vi "SentinelController v33.vi"() -> ()   [LabVIEW 2011] (continued)
                                n1665 = local write "GPIB bus 0 write error"(w1891) -> ()
                                n1666 = local write "GPIB Bus 0 traffic"(w1885) -> ()
                                }
                                }
                                frame #2 {
                                n1667 = local read "H2 loop counter hid"() -> (w1892:u32)
                                n1668 = Increment(x=w1892) -> (x+1=w1893:u32)
                                n1669 = local write "H2 loop counter hid"(w1893) -> ()
                                }
                                }
                                }
                                }
                                }
                                frame True {
                                n1670 = flat-sequence {
                                frame #0 {
                                n1671 = local write "Last locked handler hid"(enum16{"H1", "H2"}."H1" ("Last locked handler")) -> ()
                                }
                                frame #1 {
                                n1672 = while {
                                stop <- w1895 stop-if-true
                                n1673 = local read "VISA bus 0 resource name out hid"() -> (w1904:refnum<visa-resource-name>)
                                n1674 = local read "H1 SITES? response hid"() -> (w1898:string)
                                n1675 = local read "VISA bus 0 error out hid"() -> (w1905:errorcluster)
                                n1676 = VISA Write(VISA resource name=w1904, write buffer=w1898, error in (no error)=w1905) -> (VISA resource name out=w1903:refnum<visa-resource-name>, return count=w1896:u32, error out=w1902:errorcluster)
                                n1677 = local write "VISA bus 0 resource name out hid"(w1903) -> ()
                                n1678 = local write "VISA bus 0 error out hid"(w1902) -> ()
                                n1679 = Unbundle By Name(w1902) -> ("status"=w1906:bool)
                                n1680 = Concatenate Strings("H1: Tester test cycle start" ("string"), "\r\n", "Bus 0 write: " ("string"), w1898) -> (w1900:string)
                                n1681 = Greater Than 0?(x=w1896) -> (x > 0?=w1895:bool)
                                n1682 = local write "GPIB bus 0 write error"(w1906) -> ()
                                n1683 = local write "GPIB Bus 0 traffic"(w1900) -> ()
                                }
                                }
                                frame #2 {
                                n1684 = local read "H1 loop counter hid"() -> (w1908:u32)
                                n1685 = Increment(x=w1908) -> (x+1=w1907:u32)
                                n1686 = local write "H1 loop counter hid"(w1907) -> ()
                                }
                                }
                                }
                                }
                                }
                                }
                                }
                                frame #2 {
                                n1687 = Tick Count (ms)() -> (millisecond timer value=w1911:u32)
                                n1688 = Tick Count (ms)() -> (millisecond timer value=w1912:u32)
                                n1689 = local write "tester tt start hid"(w1911) -> ()
                                n1690 = local write "tester wt end hid"(w1912) -> ()
                                }
                                frame #3 {
                                n1691 = local read "tester wt start hid"() -> (w1916:u32)
                                n1692 = local read "tester wt end hid"() -> (w1917:u32)
                                n1693 = Subtract(x=w1917, y=w1916) -> (x-y=w1915:u32)
                                n1694 = Divide(x=w1915, y=u32 1000) -> (x/y=w1913:dbl)
                                n1695 = local write "SC measured wait time hid"(w1913) -> ()
                                }
                                frame #4 {
                                n1696 = local write "SC handler states hid"(SC_handler_states."testing" ("SC Test Interface States")) -> ()
                                }
                                }
                                }
                                }
                              }
                              frame "testing" {
                                n1697 = flat-sequence {
                                frame #0 {
                                # "Why not just go back to \"waiting on event\" state?  BEcause the state machine needs\nto sequence to a \"testing state\" so that the user knows where the program is and\nso that the monitor can show this as the current state... which is what it is.  So\nthis state is equivalent to the \"waiting on event\" state.  It is just called \"testing.\"\nA binning event will exit this state and take it to the \"reading\" state."
                                }
                                frame #1 {
                                n1698 = local read "VISA bus 0 resource name out hid"() -> (w1929:refnum<visa-resource-name>)
                                n1699 = local read "VISA bus 0 error out hid"() -> (w1928:errorcluster)
                                n1700 = local read "GPIB wait timeout hid"() -> (w1925:u32)
                                n1701 = VISA Wait on Event(7:w1925, 8:w1928, 11:w1929) -> (0:w1926:errorcluster, 3:w1927:refnum<visa-resource-name>)  [unwired: 2 in, 2 out]
                                n1702 = local write "VISA bus 0 resource name out hid"(w1927) -> ()
                                n1703 = local write "VISA bus 0 error out hid"(w1926) -> ()
                                }
                                frame #2 {
                                n1704 = local read "Tester loop counter hid"() -> (w1930:u32)
                                n1705 = Increment(x=w1930) -> (x+1=w1931:u32)
                                n1706 = local write "Tester loop counter hid"(w1931) -> ()
                                }
                                frame #3 {
                                n1707 = local write "SC handler states hid"(SC_handler_states."reading" ("SC Test Interface States")) -> ()
                                }
                                }
                              }
                              frame "responding to A BIN" {
                                n1708 = flat-sequence {
                                frame #0 {
                                n1709 = local read "H1 Lock"() -> (w1935:bool)
                                n1710 = case shown="False" w1935 {
                                frame False {
                                n1711 = local read "H2 Lock"() -> (w1936:bool)
                                n1712 = case shown="True" w1936 {
                                frame False {
                                }
                                frame True {
                                n1713 = local read "GPIB Bus 0 traffic"() -> (w1940:string)
                                n1714 = Concatenate Strings(w1940, "\r\n", "Bus 0: binning, calulating\ntest time, financials, releasing\nH2 lock." ("string")) -> (w1938:string)
                                n1715 = local write "GPIB Bus 0 traffic"(w1938) -> ()
                                }
                                }
                                }
                                frame True {
                                n1716 = local read "GPIB Bus 0 traffic"() -> (w1944:string)
                                n1717 = Concatenate Strings(w1944, "\r\n", "Bus 0: binning, calulating\ntest time, financials, releasing\nH1 lock." ("string")) -> (w1942:string)
                                n1718 = local write "GPIB Bus 0 traffic"(w1942) -> ()
                                }
                                }
                                }
                                frame #1 {
                                n1719 = Tick Count (ms)() -> (millisecond timer value=w1946:u32)
                                n1720 = Tick Count (ms)() -> (millisecond timer value=w1945:u32)
                                n1721 = local write "tester tt end hid"(w1946) -> ()
                                n1722 = local write "tester wt start hid"(w1945) -> ()
                                }
                                frame #2 {
                                n1723 = local read "tester tt start hid"() -> (w1950:u32)
                                n1724 = local read "tester tt end hid"() -> (w1951:u32)
                                n1725 = Subtract(x=w1951, y=w1950) -> (x-y=w1949:u32)
                                n1726 = Divide(x=w1949, y=u32 1000) -> (x/y=w1947:dbl)
                                n1727 = local write "SC measured test time hid"(w1947) -> ()
                                }
                                frame #3 {
                                n1728 = local read "H1 Lock"() -> (w1952:bool)
                                n1729 = case shown="True" w1952 {
                                frame False {
                                n1730 = local read "H2 Lock"() -> (w1953:bool)
                                n1731 = case shown="True" w1953 {
                                frame False {
                                n1732 = One Button Dialog(message="Fatal error 202:\nThe SC responded to a handler being ready with devices\nto test, but when the SC received binning data, no handler had a lock. \nPlease report this bug to Celerint at www.celerint.com  ") -> ()  [unwired: 1 in, 1 out]
                                }
                                frame True {
                                n1733 = local read "H2 online"() -> (w1974:bool)
                                n1734 = local read "Tandem\nfloorspace area"() -> (w1957:i32)
                                n1735 = local read "Std cell \nfloorspace area"() -> (w1985:i32)
                                n1736 = case shown="True" w1974 {
                                tunnel: [0 w1989] -> w1975
                                frame False {
                                }
                                frame True {
                                n1737 = local read "H2 UPH"() -> (w1990:cluster{u32, u32})
                                n1738 = Unbundle(w1990) -> (w1989:u32)  [unwired: 1 out]
                                }
                                }
                                n1739 = local read "System UPH"() -> (w1956:u32)
                                n1740 = local read "UPH"() -> (w1986:dbl)
                                n1741 = Divide(x=w1956, y=w1957) -> (x/y=w1955:dbl)
                                n1742 = local write "Tandem UPH\nper unit area"(w1955) -> ()
                                n1743 = Divide(x=w1986, y=w1985) -> (x/y=w1987:dbl)
                                n1744 = local read "Std hourly\ncost ($/hr)"() -> (w1982:dbl)
                                n1745 = local read "H1 UPH"() -> (w1984:cluster{u32, u32})
                                n1746 = local write "H1 UPH per unit area"(w1987) -> ()
                                n1747 = local read "Utilization (%)"() -> (w1967:u32)
                                n1748 = local read "Tandem hourly\ncost ($/hr)"() -> (w1983:dbl)
                                n1749 = local read "# of devices to test"() -> (w1973:u32)
                                n1750 = Unbundle(w1984) -> (w1976:u32)  [unwired: 1 out]
                                n1751 = local read "Hours per month"() -> (w1968:i32)
                                n1752 = local write "Calc H2 UPH"(w1975) -> ()
                                n1753 = local write "Calc H1 UPH"(w1976) -> ()
                                n1754 = local read "UPH"() -> (w1981:dbl)
                                n1755 = Add(x=w1976, y=w1975) -> (x+y=w1963:u32)
                                n1756 = Divide(x=w1967, y=u32 100) -> (x/y=w1966:dbl)
                                n1757 = Divide(x=w1973, y=w1963) -> (x/y=w1972:dbl)
                                n1758 = Multiply(x=w1968, y=w1966) -> (x*y=w1964:dbl)
                                n1759 = Divide(x=w1982, y=w1981) -> (x/y=w1980:dbl)
                                n1760 = Divide(x=w1983, y=w1963) -> (x/y=w1978:dbl)
                                n1761 = local write "System UPH"(w1963) -> ()
                                n1762 = local write "Calc\nsystem UPH"(w1963) -> ()
                                n1763 = local read "# of devices to test"() -> (w1961:u32)
                                n1764 = Divide(x=w1972, y=w1964) -> (x/y=w1971:dbl)
                                n1765 = Multiply(x=w1980, y=100.0) -> (x*y=w1959:dbl)
                                n1766 = Multiply(x=w1978, y=100.0) -> (x*y=w1958:dbl)
                                n1767 = local write "Std unit cost\n(cents/device)"(w1959) -> ()
                                n1768 = local write "Tandem unit cost\n(cents/device)"(w1958) -> ()
                                n1769 = Subtract(x=w1959, y=w1958) -> (x-y=w1962:dbl)
                                n1770 = Multiply(x=w1971, y=30) -> (x*y=w1969:dbl)
                                n1771 = Multiply(x=w1961, y=w1962) -> (x*y=w1960:dbl)
                                n1772 = local write "Calendar days required\nfor testing all units"(w1969) -> ()
                                n1773 = local write "$ saved"(w1960) -> ()
                                }
                                }
                                }
                                frame True {
                                n1774 = local read "H1 online"() -> (w2011:bool)
                                n1775 = local read "Tandem\nfloorspace area"() -> (w2023:i32)
                                n1776 = local read "Std cell \nfloorspace area"() -> (w2016:i32)
                                n1777 = case shown="True" w2011 {
                                tunnel: [0 w2025] -> w1991
                                frame False {
                                }
                                frame True {
                                n1778 = local read "H1 UPH"() -> (w2026:cluster{u32, u32})
                                n1779 = Unbundle(w2026) -> (w2025:u32)  [unwired: 1 out]
                                }
                                }
                                n1780 = local read "System UPH"() -> (w2022:u32)
                                n1781 = local read "H2 calc UPH"() -> (w2017:dbl)
                                n1782 = Divide(x=w2022, y=w2023) -> (x/y=w1994:dbl)
                                n1783 = Divide(x=w2017, y=w2016) -> (x/y=w1995:dbl)
                                n1784 = local write "Tandem UPH\nper unit area"(w1994) -> ()
                                n1785 = local write "H2 UPH per unit area"(w1995) -> ()
                                n1786 = local read "Std hourly\ncost ($/hr)"() -> (w2019:dbl)
                                n1787 = local read "H2 UPH"() -> (w2021:cluster{u32, u32})
                                n1788 = local read "Utilization (%)"() -> (w2001:u32)
                                n1789 = local read "Tandem hourly\ncost ($/hr)"() -> (w2020:dbl)
                                n1790 = local read "# of devices to test"() -> (w2007:u32)
                                n1791 = local read "Hours per month"() -> (w2002:i32)
                                n1792 = Unbundle(w2021) -> (w1997:u32)  [unwired: 1 out]
                                n1793 = local write "Calc H1 UPH"(w1991) -> ()
                                n1794 = local write "Calc H2 UPH"(w1997) -> ()
                                n1795 = local read "UPH"() -> (w2018:dbl)
                                n1796 = Add(x=w1991, y=w1997) -> (x+y=w1996:u32)
                                n1797 = Divide(x=w2001, y=u32 100) -> (x/y=w2000:dbl)
                                n1798 = local write "System UPH"(w1996) -> ()
                                n1799 = local write "Calc\nsystem UPH"(w1996) -> ()
                                n1800 = Divide(x=w2007, y=w1996) -> (x/y=w2006:dbl)
                                n1801 = Multiply(x=w2002, y=w2000) -> (x*y=w1998:dbl)
                                n1802 = Divide(x=w2019, y=w2018) -> (x/y=w2015:dbl)
                                n1803 = Divide(x=w2020, y=w1996) -> (x/y=w2013:dbl)
                                n1804 = local read "# of devices to test"() -> (w2009:u32)
                                n1805 = Divide(x=w2006, y=w1998) -> (x/y=w2005:dbl)
                                n1806 = Multiply(x=w2015, y=100.0) -> (x*y=w1993:dbl)
                                n1807 = Multiply(x=w2013, y=100.0) -> (x*y=w1992:dbl)
                                n1808 = local write "Std unit cost\n(cents/device)"(w1993) -> ()
                                n1809 = local write "Tandem unit cost\n(cents/device)"(w1992) -> ()
                                n1810 = Subtract(x=w1993, y=w1992) -> (x-y=w2010:dbl)
                                n1811 = Multiply(x=w2005, y=30) -> (x*y=w2003:dbl)
                                n1812 = Multiply(x=w2009, y=w2010) -> (x*y=w2008:dbl)
                                n1813 = local write "Calendar days required\nfor testing all units"(w2003) -> ()
                                n1814 = local write "$ saved"(w2008) -> ()
                                }
                                }
                                }
                                frame #4 {
                                # "when this loop unlocks the handlers,\nthe handler interface loops are free to continue\nto send the binning information to their\nrespective handlers.  Each handler interface \nloop using the \"binning string hidden\" to do\nthis.  That is why, here, there is no writing of\nthe binning informatrion to a handler.  \nThat is done in the handler interface loops."
                                n1815 = local write "H1 Lock"(FALSE ("H1 Lock")) -> ()
                                n1816 = local write "H2 Lock"(FALSE ("H1 Lock")) -> ()
                                }
                                frame #5 {
                                n1817 = local read "Tester online"() -> (w2029:bool)
                                n1818 = local read "POWER"() -> (w2031:bool)
                                n1819 = Compound Arithmetic op=AND(w2029, w2031) -> (w2030:bool)
                                n1820 = case shown="True" w2030 {
                                frame False {
                                n1821 = local write "SC handler states hid"(SC_handler_states."closing bus" ("SC virtual handler states")) -> ()
                                }
                                frame True {
                                n1822 = local write "SC handler states hid"(SC_handler_states."waiting on event" ("SC virtual handler states")) -> ()
                                }
                                }
                                }
                                }
                              }
                              frame "responding to BINON" {
                                n1823 = local read "H1 Lock"() -> (w2034:bool)
                                n1824 = case shown="True" w2034 {
                                frame False {
                                n1825 = local read "H2 Lock"() -> (w2037:bool)
                                n1826 = case shown="True" w2037 {
                                frame False {
                                }
                                frame True {
                                n1827 = flat-sequence {
                                frame #0 {
                                n1828 = local read "H2 echo hid"() -> (w2038:string)
                                n1829 = local read "VISA bus 0 resource name out hid"() -> (w2047:refnum<visa-resource-name>)
                                n1830 = local read "VISA bus 0 error out hid"() -> (w2046:errorcluster)
                                n1831 = local read "GPIB Bus 0 traffic"() -> (w2043:string)
                                n1832 = VISA Write(VISA resource name=w2047, write buffer=w2038, error in (no error)=w2046) -> (VISA resource name out=w2045:refnum<visa-resource-name>, error out=w2044:errorcluster)  [unwired: 1 out]
                                n1833 = local write "VISA bus 0 resource name out hid"(w2045) -> ()
                                n1834 = Unbundle By Name(w2044) -> ("status"=w2039:bool)
                                n1835 = local write "VISA bus 0 error out hid"(w2044) -> ()
                                n1836 = Concatenate Strings(w2043, "\r\n", "Bus 0 write: " ("string"), w2038) -> (w2041:string)
                                n1837 = local write "GPIB Bus 0 traffic"(w2041) -> ()
                                n1838 = local write "GPIB bus 0 write error"(w2039) -> ()
                                }
                                frame #1 {
                                n1839 = local write "SC handler states hid"(SC_handler_states."waiting on event" ("SC Test Interface States")) -> ()
                                }
                                }
                                }
                                }
                                }
                                frame True {
                                n1840 = flat-sequence {
                                frame #0 {
                                n1841 = local read "H1 echo hid"() -> (w2049:string)
                                n1842 = local read "VISA bus 0 resource name out hid"() -> (w2058:refnum<visa-resource-name>)
                                n1843 = local read "VISA bus 0 error out hid"() -> (w2057:errorcluster)
                                n1844 = local read "GPIB Bus 0 traffic"() -> (w2054:string)
                                n1845 = VISA Write(VISA resource name=w2058, write buffer=w2049, error in (no error)=w2057) -> (VISA resource name out=w2056:refnum<visa-resource-name>, error out=w2055:errorcluster)  [unwired: 1 out]
                                n1846 = local write "VISA bus 0 resource name out hid"(w2056) -> ()
                                n1847 = Unbundle By Name(w2055) -> ("status"=w2050:bool)
                                n1848 = local write "VISA bus 0 error out hid"(w2055) -> ()
                                n1849 = Concatenate Strings(w2054, "\r\n", "Bus 0 write: " ("string"), w2049) -> (w2052:string)
                                n1850 = local write "GPIB Bus 0 traffic"(w2052) -> ()
                                n1851 = local write "GPIB bus 0 write error"(w2050) -> ()
                                }
                                frame #1 {
                                n1852 = local write "SC handler states hid"(SC_handler_states."waiting on event" ("SC Test Interface States")) -> ()
                                }
                                }
                                }
                                }
                              }
                              frame "responding to ECHONG" {
                                n1853 = flat-sequence {
                                frame #0 {
                                # "Echo was returned to the tester via the BINON state"
                                n1854 = local read "H1 Lock"() -> (w2062:bool)
                                n1855 = case shown="False" w2062 {
                                frame False {
                                n1856 = local read "H2 Lock"() -> (w2063:bool)
                                n1857 = case shown="True" w2063 {
                                frame False {
                                }
                                frame True {
                                n1858 = local read "GPIB Bus 0 traffic"() -> (w2067:string)
                                n1859 = Concatenate Strings(w2067, "\r\n", "Bus 0: ECHONG received for H2. Retrying." ("string")) -> (w2065:string)
                                n1860 = local write "GPIB Bus 0 traffic"(w2065) -> ()
                                }
                                }
                                }
                                frame True {
                                n1861 = local read "GPIB Bus 0 traffic"() -> (w2071:string)
                                n1862 = Concatenate Strings(w2071, "\r\n", "Bus 0: ECHONG received for H1. Retrying." ("string")) -> (w2069:string)
                                n1863 = local write "GPIB Bus 0 traffic"(w2069) -> ()
                                }
                                }
                                }
                                frame #1 {
                                n1864 = local write "SC handler states hid"(SC_handler_states."waiting on event" ("SC Test Interface States")) -> ()
                                }
                                }
                              }
                              frame "responding to ECHOOK" {
                                n1865 = flat-sequence {
                                frame #0 {
                                # "Echo was returned to the tester via the BINON state"
                                n1866 = local read "H1 Lock"() -> (w2075:bool)
                                n1867 = case shown="True" w2075 {
                                frame False {
                                n1868 = local read "H2 Lock"() -> (w2076:bool)
                                n1869 = case shown="False" w2076 {
                                frame False {
                                }
                                frame True {
                                n1870 = local read "GPIB Bus 0 traffic"() -> (w2080:string)
                                n1871 = Concatenate Strings(w2080, "\r\n", "Bus 0: ECHOOK received for H2.\nCalculating test time, financials,\nreleasing H2 Lock." ("string")) -> (w2078:string)
                                n1872 = local write "GPIB Bus 0 traffic"(w2078) -> ()
                                }
                                }
                                }
                                frame True {
                                n1873 = local read "GPIB Bus 0 traffic"() -> (w2084:string)
                                n1874 = Concatenate Strings(w2084, "\r\n", "Bus 0: ECHOOK received for H1.\nCalculating test time, financials,\nreleasing H1 Lock." ("string")) -> (w2082:string)
                                n1875 = local write "GPIB Bus 0 traffic"(w2082) -> ()
                                }
                                }
                                }
                                frame #1 {
                                n1876 = Tick Count (ms)() -> (millisecond timer value=w2086:u32)
                                n1877 = Tick Count (ms)() -> (millisecond timer value=w2085:u32)
                                n1878 = local write "tester tt end hid"(w2086) -> ()
                                n1879 = local write "tester wt start hid"(w2085) -> ()
                                }
                                frame #2 {
                                n1880 = local read "tester tt start hid"() -> (w2090:u32)
                                n1881 = local read "tester tt end hid"() -> (w2091:u32)
                                n1882 = Subtract(x=w2091, y=w2090) -> (x-y=w2089:u32)
                                n1883 = Divide(x=w2089, y=u32 1000) -> (x/y=w2087:dbl)
                                n1884 = local write "SC measured test time hid"(w2087) -> ()
                                }
                                frame #3 {
                                n1885 = local read "H1 Lock"() -> (w2092:bool)
                                n1886 = case shown="True" w2092 {
                                frame False {
                                n1887 = local read "H2 Lock"() -> (w2093:bool)
                                n1888 = case shown="True" w2093 {
                                frame False {
                                n1889 = One Button Dialog(message="Fatal error 202:\nThe SC responded to a handler being ready with devices\nto test, but when the SC received binning data, no handler had a lock. \nPlease report this bug to Celerint at www.celerint.com  ") -> ()  [unwired: 1 in, 1 out]
                                }
                                frame True {
                                n1890 = local read "H2 online"() -> (w2114:bool)
                                n1891 = local read "Tandem\nfloorspace area"() -> (w2097:i32)
                                n1892 = local read "Std cell \nfloorspace area"() -> (w2125:i32)
                                n1893 = case shown="True" w2114 {
                                tunnel: [0 w2129] -> w2115
                                frame False {
                                }
                                frame True {
                                n1894 = local read "H2 UPH"() -> (w2130:cluster{u32, u32})
                                n1895 = Unbundle(w2130) -> (w2129:u32)  [unwired: 1 out]
                                }
                                }
                                n1896 = local read "System UPH"() -> (w2096:u32)
                                n1897 = local read "UPH"() -> (w2126:dbl)
                                n1898 = Divide(x=w2096, y=w2097) -> (x/y=w2095:dbl)
                                n1899 = local write "Tandem UPH\nper unit area"(w2095) -> ()
                                n1900 = Divide(x=w2126, y=w2125) -> (x/y=w2127:dbl)
                                n1901 = local read "Std hourly\ncost ($/hr)"() -> (w2122:dbl)
                                n1902 = local read "H1 UPH"() -> (w2124:cluster{u32, u32})
                                n1903 = local write "H1 UPH per unit area"(w2127) -> ()
                                n1904 = local read "Utilization (%)"() -> (w2107:u32)
                                n1905 = local read "Tandem hourly\ncost ($/hr)"() -> (w2123:dbl)
                                n1906 = local read "# of devices to test"() -> (w2113:u32)
                                n1907 = Unbundle(w2124) -> (w2116:u32)  [unwired: 1 out]
                                n1908 = local read "Hours per month"() -> (w2108:i32)
                                n1909 = local write "Calc H2 UPH"(w2115) -> ()
                                n1910 = local write "Calc H1 UPH"(w2116) -> ()
                                n1911 = local read "UPH"() -> (w2121:dbl)
                                n1912 = Add(x=w2116, y=w2115) -> (x+y=w2103:u32)
                                n1913 = Divide(x=w2107, y=u32 100) -> (x/y=w2106:dbl)
                                n1914 = Divide(x=w2113, y=w2103) -> (x/y=w2112:dbl)
                                n1915 = Multiply(x=w2108, y=w2106) -> (x*y=w2104:dbl)
                                n1916 = Divide(x=w2122, y=w2121) -> (x/y=w2120:dbl)
                                n1917 = Divide(x=w2123, y=w2103) -> (x/y=w2118:dbl)
                                n1918 = local write "System UPH"(w2103) -> ()
                                n1919 = local write "Calc\nsystem UPH"(w2103) -> ()
                                n1920 = local read "# of devices to test"() -> (w2101:u32)
                                n1921 = Divide(x=w2112, y=w2104) -> (x/y=w2111:dbl)
                                n1922 = Multiply(x=w2120, y=100.0) -> (x*y=w2099:dbl)
                                n1923 = Multiply(x=w2118, y=100.0) -> (x*y=w2098:dbl)
                                n1924 = local write "Std unit cost\n(cents/device)"(w2099) -> ()
                                n1925 = local write "Tandem unit cost\n(cents/device)"(w2098) -> ()
                                n1926 = Subtract(x=w2099, y=w2098) -> (x-y=w2102:dbl)
                                n1927 = Multiply(x=w2111, y=30) -> (x*y=w2109:dbl)
                                n1928 = Multiply(x=w2101, y=w2102) -> (x*y=w2100:dbl)
                                n1929 = local write "Calendar days required\nfor testing all units"(w2109) -> ()
                                n1930 = local write "$ saved"(w2100) -> ()
                                }
                                }
                                }
                                frame True {
                                n1931 = local read "H1 online"() -> (w2151:bool)
                                n1932 = local read "Tandem\nfloorspace area"() -> (w2163:i32)
                                n1933 = local read "Std cell \nfloorspace area"() -> (w2156:i32)
                                n1934 = case shown="True" w2151 {
                                tunnel: [0 w2165] -> w2131
                                frame False {
                                }
                                frame True {
                                n1935 = local read "H1 UPH"() -> (w2166:cluster{u32, u32})
                                n1936 = Unbundle(w2166) -> (w2165:u32)  [unwired: 1 out]
                                }
                                }
                                n1937 = local read "System UPH"() -> (w2162:u32)
                                n1938 = local read "H2 calc UPH"() -> (w2157:dbl)
                                n1939 = Divide(x=w2162, y=w2163) -> (x/y=w2134:dbl)
                                n1940 = Divide(x=w2157, y=w2156) -> (x/y=w2135:dbl)
                                n1941 = local write "Tandem UPH\nper unit area"(w2134) -> ()
                                n1942 = local write "H2 UPH per unit area"(w2135) -> ()
                                n1943 = local read "Std hourly\ncost ($/hr)"() -> (w2159:dbl)
                                n1944 = local read "H2 UPH"() -> (w2161:cluster{u32, u32})
                                n1945 = local read "Utilization (%)"() -> (w2141:u32)
                                n1946 = local read "Tandem hourly\ncost ($/hr)"() -> (w2160:dbl)
                                n1947 = local read "# of devices to test"() -> (w2147:u32)
                                n1948 = local read "Hours per month"() -> (w2142:i32)
                                n1949 = Unbundle(w2161) -> (w2137:u32)  [unwired: 1 out]
                                n1950 = local write "Calc H1 UPH"(w2131) -> ()
                                n1951 = local write "Calc H2 UPH"(w2137) -> ()
                                n1952 = local read "UPH"() -> (w2158:dbl)
                                n1953 = Add(x=w2131, y=w2137) -> (x+y=w2136:u32)
                                n1954 = Divide(x=w2141, y=u32 100) -> (x/y=w2140:dbl)
                                n1955 = local write "System UPH"(w2136) -> ()
                                n1956 = local write "Calc\nsystem UPH"(w2136) -> ()
                                n1957 = Divide(x=w2147, y=w2136) -> (x/y=w2146:dbl)
                                n1958 = Multiply(x=w2142, y=w2140) -> (x*y=w2138:dbl)
                                n1959 = Divide(x=w2159, y=w2158) -> (x/y=w2155:dbl)
                                n1960 = Divide(x=w2160, y=w2136) -> (x/y=w2153:dbl)
                                n1961 = local read "# of devices to test"() -> (w2149:u32)
                                n1962 = Divide(x=w2146, y=w2138) -> (x/y=w2145:dbl)
                                n1963 = Multiply(x=w2155, y=100.0) -> (x*y=w2133:dbl)
                                n1964 = Multiply(x=w2153, y=100.0) -> (x*y=w2132:dbl)
                                n1965 = local write "Std unit cost\n(cents/device)"(w2133) -> ()
                                n1966 = local write "Tandem unit cost\n(cents/device)"(w2132) -> ()
                                n1967 = Subtract(x=w2133, y=w2132) -> (x-y=w2150:dbl)
                                n1968 = Multiply(x=w2145, y=30) -> (x*y=w2143:dbl)
                                n1969 = Multiply(x=w2149, y=w2150) -> (x*y=w2148:dbl)
                                n1970 = local write "Calendar days required\nfor testing all units"(w2143) -> ()
                                n1971 = local write "$ saved"(w2148) -> ()
                                }
                                }
                                }
                                frame #4 {
                                # "when this loop unlocks the handlers,\nthe handler interface loops are free to continue\nto send the binning information to their\nrespective handlers.  Each handler interface \nloop using the \"binning string hidden\" to do\nthis.  That is why, here, there is no writing of\nthe binning informatrion to a handler.  \nThat is done in the handler interface loops."
                                n1972 = local write "H1 Lock"(FALSE ("H1 Lock")) -> ()
                                n1973 = local write "H2 Lock"(FALSE ("H1 Lock")) -> ()
                                }
                                frame #5 {
                                n1974 = local read "Tester online"() -> (w2169:bool)
                                n1975 = local read "POWER"() -> (w2171:bool)
                                n1976 = Compound Arithmetic op=AND(w2169, w2171) -> (w2170:bool)
                                n1977 = case shown="False" w2170 {
                                frame False {
                                n1978 = local write "SC handler states hid"(SC_handler_states."closing bus" ("SC virtual handler states")) -> ()
                                }
                                frame True {
                                n1979 = local write "SC handler states hid"(SC_handler_states."waiting on serial poll" ("SC Test Interface States")) -> ()
                                }
                                }
                                }
                                }
                              }
                              frame "closing bus" {
                                n1980 = flat-sequence {
                                frame #0 {
                                n1981 = local read "GPIB Bus 0 traffic"() -> (w2179:string)
                                n1982 = Concatenate Strings(w2179, "\r\n", "Bus 0 closing: " ("string")) -> (w2177:string)
                                n1983 = local write "GPIB Bus 0 traffic"(w2177) -> ()
                                }
                                frame #1 {
                                n1984 = local read "VISA bus 0 resource name out hid"() -> (w2181:refnum<visa-resource-name>)
                                n1985 = local read "VISA bus 0 error out hid"() -> (w2182:errorcluster)
                                n1986 = VISA Close(VISA resource name=w2181, error in (no error)=w2182) -> (error out=w2180:errorcluster)
                                n1987 = Unbundle By Name(w2180) -> ("status"=w2183:bool)
                                n1988 = local write "VISA bus 0 close error"(w2183) -> ()
                                }
                                frame #2 {
                                n1989 = local write "Exit SC handler StMach hid"(TRUE ("Exit tester state machine hid")) -> ()
                                }
                                }
                              }
                              frame "responding to unknown command" {
                                n1990 = flat-sequence {
                                frame #0 {
                                n1991 = local read "GPIB Bus 0 traffic"() -> (w2191:string)
                                n1992 = Concatenate Strings(w2191, "\r\n", "Bus 0 write: " ("string"), "unrecognized string") -> (w2189:string)
                                n1993 = local write "GPIB Bus 0 traffic"(w2189) -> ()
                                }
                                frame #1 {
                                n1994 = local write "SC handler states hid"(SC_handler_states."waiting on event" ("SC Test Interface States")) -> ()
                                }
                                }
                              }
                            }
                          }
                          frame #1 {
                            n1995 = local read "Slow for  Diagnostics"() -> (w2193:bool)
                            n1996 = case shown="True" w2193 {
                              frame False {
                              }
                              frame True {
                                n1997 = local read "GPIB wait time (ms)"() -> (w2196:u32)
                                n1998 = Wait (ms)(milliseconds to wait=w2196) -> ()  [unwired: 1 out]
                              }
                            }
                          }
                        }
                        n1999 = Wait (ms)(milliseconds to wait=u32 1) -> ()  [unwired: 1 out]
                        n2000 = local read "Exit SC handler StMach hid"() -> (w1380:bool)
                        "Numeric" <- w1376
                      }
                    }
                  }
                }
              }
              n2001 = Wait (ms)(milliseconds to wait=u32 5) -> ()  [unwired: 1 out]
              n2002 = local read "POWER"() -> (w1366:bool)
            }
            n2003 = while {
              stop <- w360 continue-if-true
              n2004 = local read "H1 online"() -> (w361:bool)
              n2005 = case shown="True" w361 {
                frame False {
                }
                frame True {
                  n2006 = flat-sequence {
                    frame #0 {
                      n2007 = local write "Exit SC tester H1 StMach hid"(FALSE ("Exit H1 state machine hid")) -> ()
                    }
                    frame #1 {
                      n2008 = local read "H1 handler type"() -> (w363:T2)
                      n2009 = case shown="\"Seiko-Epson NS6040\"" w363 {
                        frame "Multitest", Default {
                          n2010 = local write "MT99XX tester states H1 hid"(SC_MT99XX_tester_states."initializing bus" ("SC virtual tester states")) -> ()
                          n2011 = flat-sequence {
                            frame #0 {
                              n2012 = local read "MT99XX tester states H1 hid"() -> (w365:T4)
                              n2013 = case shown="\"binning\"" w365 {
                                frame "initializing bus", Default {
                                n2014 = flat-sequence {
                                frame #0 {
                                # "bus 1"
                                n2015 = local read "GPIB wait timeout hid"() -> (w369:u32)
                                n2016 = local read "SentCtrl talks to handler 1 at"() -> (w370:refnum<visa-resource-name>)
                                n2017 = local read "GPIB wait timeout hid"() -> (w368:u32)
                                n2018 = VISA Open(timeout (0)=w369, VISA resource name=w370) -> (VISA resource name=w367:refnum<visa-resource-name>, error out=w372:errorcluster)  [unwired: 3 in]
                                n2019 = property class="GPIB Instr"(reference=w367, error in=w372, "Timeout"=w368) -> (error out=w366:errorcluster)  [unwired: 1 out]
                                n2020 = local write "VISA bus 1 resource name out hid"(w367) -> ()
                                n2021 = Unbundle By Name(w366) -> ("status"=w371:bool)
                                n2022 = local write "VISA bus 1 open error"(w371) -> ()
                                n2023 = local write "VISA bus 1 error out hid"(w366) -> ()
                                }
                                frame #1 {
                                n2024 = local write "Exit SC tester H1 StMach hid"(FALSE ("Exit H1 state machine hid")) -> ()
                                n2025 = Concatenate Strings("Bus 1 initializing" ("string"), "\r\n") -> (w375:string)
                                n2026 = local write "GPIB bus 1 traffic"(w375) -> ()
                                }
                                frame #2 {
                                n2027 = local write "MT99XX tester states H1 hid"(SC_MT99XX_tester_states."sending *IDN?" ("SC virtual tester states")) -> ()
                                }
                                }
                                }
                                frame "sending *IDN?" {
                                n2028 = flat-sequence {
                                tunnel: [w387] -> w380
                                tunnel: [w386] -> w379
                                tunnel: w380 -> [w401]
                                tunnel: w379 -> [w400]
                                tunnel: [w391] -> w378
                                tunnel: w378 -> [w402]
                                frame #0 {
                                w381 = "*IDN?"
                                n2029 = local read "VISA bus 1 resource name out hid"() -> (w390:refnum<visa-resource-name>)
                                n2030 = local read "GPIB bus 1 traffic"() -> (w385:string)
                                n2031 = local read "VISA bus 1 error out hid"() -> (w389:errorcluster)
                                n2032 = Concatenate Strings(w385, "\r\n", "Bus 1 write: " ("string"), w381) -> (w383:string)
                                n2033 = VISA Write(VISA resource name=w390, write buffer=w381, error in (no error)=w389) -> (VISA resource name out=w387:refnum<visa-resource-name>, error out=w386:errorcluster)  [unwired: 1 out]
                                n2034 = Unbundle By Name(w386) -> ("status"=w388:bool)
                                n2035 = local write "GPIB bus 1 traffic"(w383) -> ()
                                n2036 = local write "GPIB bus 1 write error"(w388) -> ()
                                }
                                frame #1 {
                                n2037 = local read "GPIB bus 1 traffic"() -> (w393:string)
                                n2038 = VISA Read(VISA resource name=w401, byte count=u32 256, error in (no error)=w400) -> (VISA resource name out=w398:refnum<visa-resource-name>, read buffer=w392:string, error out=w397:errorcluster)  [unwired: 1 out]
                                n2039 = local write "VISA bus 1 resource name out hid"(w398) -> ()
                                n2040 = Unbundle By Name(w397) -> ("status"=w391:bool)
                                n2041 = local write "H1 response to *IDN? hid"(w392) -> ()
                                n2042 = local write "GPIB bus 1 read error"(w391) -> ()
                                n2043 = Concatenate Strings(w393, "\r\n", "Bus 1 read: " ("string"), w392) -> (w395:string)
                                n2044 = local write "GPIB bus 1 traffic"(w395) -> ()
                                }
                                frame #2 {
                                n2045 = case shown="False" w402 {
                                frame False {
                                n2046 = local write "MT99XX tester states H1 hid"(SC_MT99XX_tester_states."polling *SITES?" ("SC virtual tester states")) -> ()
                                }
                                frame True {
                                n2047 = flat-sequence {
                                frame #0 {
                                n2048 = while {
                                stop <- w405 stop-if-true
                                n2049 = One Button Dialog(message="Warning:\nVirtual tester does not get a response\nto *IDN? from handler 1.\nCheck GPIB cable and that  handler 1 \nis running and ready to issue a start of test\nby responding with sites ready.", button name ("OK")="Dismiss and retry") -> (true=w405:bool)
                                n2050 = Wait (ms)(milliseconds to wait=u32 100) -> ()  [unwired: 1 out]
                                }
                                }
                                frame #1 {
                                n2051 = local write "H1 online"(FALSE ("H1 online")) -> ()
                                }
                                frame #2 {
                                n2052 = local write "MT99XX tester states H1 hid"(SC_MT99XX_tester_states."sending *IDN?" ("SC virtual tester states")) -> ()
                                }
                                }
                                }
                                }
                                }
                                }
                                }
                                frame "polling *SITES?" {
                                n2053 = flat-sequence {
                                tunnel: [w413] -> w411
                                tunnel: [w412] -> w410
                                tunnel: w411 -> [w449]
                                tunnel: w410 -> [w448]
                                frame #0 {
                                n2054 = while {
                                tunnel: [w417] -> w413
                                tunnel: [w415] -> w412
                                stop <- w414 stop-if-true
                                n2055 = stacked-sequence {
                                tunnel: [w429] -> w419
                                tunnel: [w428] -> w418
                                frame #0 {
                                w421 = "*SITES?"
                                n2056 = local read "VISA bus 1 resource name out hid"() -> (w427:refnum<visa-resource-name>)
                                n2057 = local read "VISA bus 1 error out hid"() -> (w426:errorcluster)
                                n2058 = Concatenate Strings("Handler 1 cycle start" ("string"), "\r\n", "Bus 1 write: " ("string"), w421) -> (w423:string)
                                n2059 = VISA Write(VISA resource name=w427, write buffer=w421, error in (no error)=w426) -> (VISA resource name out=w429:refnum<visa-resource-name>, error out=w428:errorcluster)  [unwired: 1 out]
                                n2060 = Unbundle By Name(w428) -> ("status"=w425:bool)
                                n2061 = local write "GPIB bus 1 traffic"(w423) -> ()
                                n2062 = local write "GPIB bus 1 write error"(w425) -> ()
                                }
                                }
                                n2063 = Wait (ms)(milliseconds to wait=u32 1) -> ()  [unwired: 1 out]
                                n2064 = flat-sequence {
                                tunnel: w419 -> [w447]
                                tunnel: w418 -> [w446]
                                tunnel: [w434] -> w417
                                tunnel: [w430] -> w415
                                tunnel: [w431] -> w414
                                frame #0 {
                                n2065 = local read "GPIB bus 1 traffic"() -> (w439:string)
                                n2066 = VISA Read(VISA resource name=w447, byte count=u32 256, error in (no error)=w446) -> (read buffer=w434:string, error out=w433:errorcluster)  [unwired: 2 out]
                                n2067 = Unbundle By Name(w433) -> ("status"=w430:bool)
                                n2068 = String Length(string=w434) -> (length=w436:i32)
                                n2069 = Scan Value(string=w434, format string="%b", default (0 dbl)=u8 0) -> (value=w438:u8)  [unwired: 1 out]
                                n2070 = Concatenate Strings(w439, "\r\n", "Bus 1 read: " ("string"), w434) -> (w441:string)
                                n2071 = local write "GPIB bus 1 read error"(w430) -> ()
                                n2072 = Greater Than 0?(x=w436) -> (x > 0?=w435:bool)
                                n2073 = Greater Than 0?(x=w438) -> (x > 0?=w437:bool)
                                n2074 = local write "GPIB bus 1 traffic"(w441) -> ()
                                n2075 = And(x=w435, y=w437) -> (x .and. y?=w432:bool)
                                n2076 = Or(x=w432, y=w430) -> (x .or. y?=w431:bool)
                                }
                                }
                                }
                                }
                                frame #1 {
                                n2077 = case shown="False" w448 {
                                tunnel: w449 -> [w450 _]
                                frame False {
                                n2078 = flat-sequence {
                                tunnel: w450 -> [w451]
                                frame #0 {
                                n2079 = String Length(string=w451) -> (length=w452:i32)
                                n2080 = local write "H1 SITES? response hid"(w451) -> ()
                                n2081 = local write "H1 parallelism"(w452) -> ()
                                }
                                frame #1 {
                                # "This block adds zeroes (sites not ready)\nto SITES READY from handlers when the\nhandler is running at a lower parallelism\nthan the test program, but has the same\npin mapping for the active sites in common."
                                n2082 = local read "Program Parallelism"() -> (w456:u32)
                                n2083 = local read "H1 allow lower parallelism"() -> (w455:bool)
                                n2084 = local read "H1 parallelism"() -> (w457:u32)
                                n2085 = Less?(x=w457, y=w456) -> (x < y?=w454:bool)
                                n2086 = And(x=w454, y=w455) -> (x .and. y?=w453:bool)
                                n2087 = case shown="True" w453 {
                                frame False {
                                n2088 = local read "Program Parallelism"() -> (w460:u32)
                                n2089 = local read "H1 parallelism"() -> (w458:u32)
                                n2090 = Greater?(x=w458, y=w460) -> (0:w459:bool)
                                n2091 = case shown="True" w459 {
                                frame False {
                                # "parallelisms must match if arriving here"
                                n2092 = local write "MT99XX tester states H1 hid"(SC_MT99XX_tester_states."testing" ("SC virtual tester states")) -> ()
                                }
                                frame True {
                                n2093 = local write "MT99XX tester states H1 hid"(SC_MT99XX_tester_states."closing bus" ("SC virtual tester states")) -> ()
                                n2094 = local write "POWER"(FALSE ("POWER")) -> ()
                                n2095 = One Button Dialog(message="Fatal error 300:\nTest program cannot support higher\nparallelism on handler 1.\nThe Sentinel Controller program is shutting down.\nPlease correct the mismatch and restart.") -> ()  [unwired: 1 in, 1 out]
                                }
                                }
                                }
                                frame True {
                                n2096 = local read "Program Parallelism"() -> (w470:u32)
                                n2097 = local read "H1 parallelism"() -> (w467:u32)
                                n2098 = local read "H1 SITES? response hid"() -> (w468:string)
                                n2099 = Subtract(x=w470, y=w467) -> (x-y=w469:u32)
                                n2100 = for {
                                N: w469 -> [_]
                                shift-right: [w471] -> w465
                                shift-left: w468 -> [w472]
                                n2101 = Concatenate Strings(w472, "0" ("string")) -> (w471:string)
                                }
                                n2102 = local write "H1 SITES? response hid"(w465) -> ()
                                n2103 = local write "MT99XX tester states H1 hid"(SC_MT99XX_tester_states."testing" ("SC virtual tester states")) -> ()
                                }
                                }
                                }
                                frame #2 {
                                n2104 = Tick Count (ms)() -> (millisecond timer value=w478:u32)
                                n2105 = Tick Count (ms)() -> (millisecond timer value=w477:u32)
                                n2106 = local write "H1 Ready with sites"(TRUE ("H2 Waiting")) -> ()
                                n2107 = local write "H1 wt start hidden"(w478) -> ()
                                n2108 = local write "H1 it end hidden"(w477) -> ()
                                n2109 = local write "H1 Indexing"(FALSE ("h1 indexing")) -> ()
                                n2110 = local write "H1 Testing"(FALSE ("h1 indexing")) -> ()
                                }
                                frame #3 {
                                n2111 = local read "H1 it start hidden"() -> (w482:u32)
                                n2112 = local read "H1 it end hidden"() -> (w483:u32)
                                n2113 = Subtract(x=w483, y=w482) -> (x-y=w479:u32)
                                n2114 = Divide(x=w479, y=u32 1000) -> (x/y=w481:dbl)
                                n2115 = local write "MT99XX tester states H1 hid"(SC_MT99XX_tester_states."testing" ("SC virtual tester states")) -> ()
                                n2116 = local write "H1 measured Index Time"(w481) -> ()
                                }
                                }
                                }
                                frame True {
                                n2117 = flat-sequence {
                                frame #0 {
                                n2118 = local read "VISA bus 1 resource name out hid"() -> (w487:refnum<visa-resource-name>)
                                n2119 = local read "VISA bus 1 error out hid"() -> (w488:errorcluster)
                                n2120 = VISA Close(VISA resource name=w487, error in (no error)=w488) -> (error out=w486:errorcluster)
                                n2121 = Unbundle By Name(w486) -> ("status"=w485:bool)
                                n2122 = local write "VISA bus 1 close error"(w485) -> ()
                                }
                                frame #1 {
                                n2123 = local write "VISA bus 1 close error"(FALSE ("VISA bus 1 close error")) -> ()
                                n2124 = Concatenate Strings("Bus 1 error  while reading,\nclosing Bus 1 and re-initializing" ("string"), "\r\n") -> (w491:string)
                                n2125 = local write "GPIB bus 1 traffic"(w491) -> ()
                                }
                                frame #2 {
                                n2126 = local write "MT99XX tester states H1 hid"(SC_MT99XX_tester_states."initializing bus" ("SC virtual tester states")) -> ()
                                }
                                }
                                }
                                }
                                }
                                }
                                }
                                frame "testing" {
                                n2127 = flat-sequence {
                                frame #0 {
                                n2128 = while {
                                stop <- w494 stop-if-true
                                n2129 = local read "H1 Lock"() -> (w494:bool)
                                n2130 = Wait (ms)(milliseconds to wait=u32 1) -> ()  [unwired: 1 out]
                                }
                                }
                                frame #1 {
                                n2131 = Tick Count (ms)() -> (millisecond timer value=w505:u32)
                                n2132 = Tick Count (ms)() -> (millisecond timer value=w504:u32)
                                n2133 = local write "H1 Testing"(TRUE ("testing")) -> ()
                                n2134 = local write "H1 Ready with sites"(FALSE ("H1 Waiting")) -> ()
                                n2135 = local write "H1 Indexing"(FALSE ("waiting")) -> ()
                                n2136 = local write "H1 wt end hidden"(w505) -> ()
                                n2137 = local write "H1 tt start hidden"(w504) -> ()
                                n2138 = local read "GPIB bus 1 traffic"() -> (w497:string)
                                n2139 = Concatenate Strings(w497, "\r\n", "Bus 1: " ("string"), "testing" ("string")) -> (w499:string)
                                n2140 = local write "GPIB bus 1 traffic"(w499) -> ()
                                }
                                frame #2 {
                                n2141 = local read "H1 wt start hidden"() -> (w509:u32)
                                n2142 = local read "H1 wt end hidden"() -> (w510:u32)
                                n2143 = Subtract(x=w510, y=w509) -> (x-y=w508:u32)
                                n2144 = Divide(x=w508, y=u32 1000) -> (x/y=w506:dbl)
                                n2145 = local write "H1 measured Wait Time"(w506) -> ()
                                }
                                frame #3 {
                                n2146 = local write "MT99XX tester states H1 hid"(SC_MT99XX_tester_states."binning" ("SC virtual tester states")) -> ()
                                }
                                }
                                }
                                frame "binning" {
                                n2147 = flat-sequence {
                                tunnel: [w523] -> w514
                                tunnel: [w550] -> w515
                                tunnel: w514 -> [w550]
                                tunnel: w515 -> [w557]
                                tunnel: [w556] -> w513
                                tunnel: [w555] -> w512
